vi "Query Parallel Configuration.vi"(0 "VISA resource name":refnum<visa-resource-name>, 11 "error in (no error)":errorcluster) -> (4 "VISA resource name out":refnum<visa-resource-name>, 6 "Auxiliaries IP LSBs":u16[](array[numeric]), 15 "error out":errorcluster)   [LabVIEW 2012, in "NH Research Regenerative Test Series.lvlib"]
doc: "This command reads the parallel configuration. This command is only sent to the module that is the master. All modules to be paralleled with the master must be set to static IP and all must be on the same IP subnet as the master. For example, if the master IP is 192.100.27.45, then all auxiliaries must have an IP of 192.100.27.xxx.\n\nThis command uses only the last byte (least significant byte LSB) of the IP address. The auxiliaries full IP is the masters IP subnet plus the auxiliaries IP LSB."
uses:
  <instrlib>/NH Research Regenerative Test Series/NH Research Regenerative Test Series.lvlib
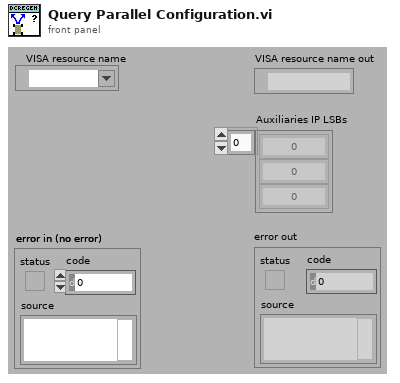
[diagram p1: front panel]
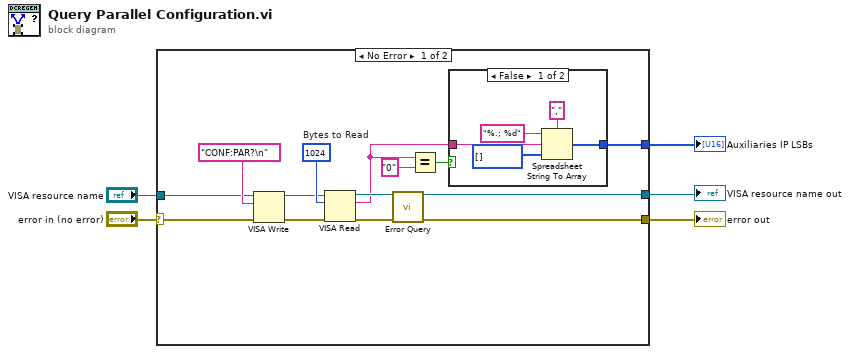
[diagram p0: block diagram]
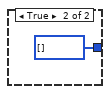
[diagram p2: hidden frame]
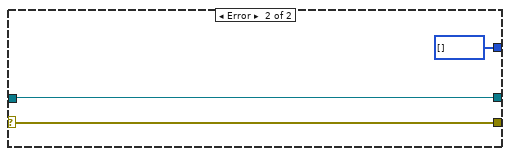
[diagram p3: hidden frame]
diagram:
  n1 = case shown="No Error" "error in (no error)" {
    selector: "error in (no error)" -> [w15 w28]
    tunnel: [w10 w28] -> w4
    tunnel: [w13 w27] -> w2
    tunnel: "VISA resource name" -> [w14 w27]
    tunnel: [w9 u16[] []] -> w1
    frame No Error {
      w19 = u32 1024  # Bytes to Read
      n2 = VISA Write(VISA resource name=w14, write buffer="CONF:PAR?\n", error in (no error)=w15) -> (VISA resource name out=w17:refnum<visa-resource-name>, error out=w18:errorcluster)  [unwired: 1 out]
      n3 = VISA Read(VISA resource name=w17, byte count=w19, error in (no error)=w18) -> (VISA resource name out=w12:refnum<visa-resource-name>, read buffer=w6:string, error out=w11:errorcluster)  [unwired: 1 out]
      n4 = call <instrlib>:"Error Query.vi"("VISA resource name"=w12, "error in (no error)"=w11) -> ("VISA resource name out"=w13:refnum<visa-resource-name>, "error out"=w10:errorcluster)  [unwired: 10 in, 2 out]
      n5 = Equal?(x=w6, y="0") -> (x = y?=w7:bool)
      n6 = case shown="False" w7 {
        tunnel: [w21 u16[] []] -> w9
        tunnel: w6 -> [w20 _]
        frame False {
          n7 = Spreadsheet String To Array(delimiter (Tab)=",", format string="%.; %d", spreadsheet string=w20, array type (2D Dbl)=u16[] []) -> (array=w21:u16[])
        }
        frame True {
        }
      }
    }
    frame Error {
    }
  }
  "error out" <- w4
  "VISA resource name out" <- w2
  "Auxiliaries IP LSBs" <- w1
